vi "ensure_selection_matches_spots.vi"(4 "Selection and Groups in":T3[](array[typedef]), 6 "Select All (default: no)":bool, 7 "Spots":T1[](array[typedef]) {"Amplitude Correction" step=0.1; "Line Trapping"."Phase Gradient" step=0.05; "Line Trapping"."Vector"."x" step=1e-06 format="%#_6p"; "Line Trapping"."Vector"."y" step=1e-06 format="%#_6p"; "Line Trapping"."Vector"."z" step=1e-06 format="%#_6p"; "NA Position"."r" step=1e-06; "NA Position"."y" step=1e-06; "NA Position"."x" step=1e-06; "Position"."z" step=1e-06; "Position"."y" step=1e-06; "Position"."x" step=1e-06; "Phase" step=0.7753; "Intensity" step=0.1}) -> (0 "Selection and Groups out":T3[](array[typedef]), 3 "Spots (duplicate)":T1[](array[typedef]) {"Amplitude Correction" step=0.1; "Line Trapping"."Phase Gradient" step=0.05; "Line Trapping"."Vector"."x" step=1e-06 format="%#_6p"; "Line Trapping"."Vector"."y" step=1e-06 format="%#_6p"; "Line Trapping"."Vector"."z" step=1e-06 format="%#_6p"; "NA Position"."r" step=1e-06; "NA Position"."y" step=1e-06; "NA Position"."x" step=1e-06; "Position"."z" step=1e-06; "Position"."y" step=1e-06; "Position"."x" step=1e-06; "Phase" step=0.7753; "Intensity" step=0.1})   [LabVIEW 2015]
doc: "This VI checks that the lengths of the \"selection\" and \"spots\" arrays are the same. If not, the selection array is replaced with a new array, having all the groups set to 0 and all the selected flags set either to true (default) or false. This can be used to ensure consistency in case of dodgy code, or to make a VI behave sensibly when the selection isn't wired in."
uses:
  spot.ctl
  line_trapping.ctl
  selection_element.ctl
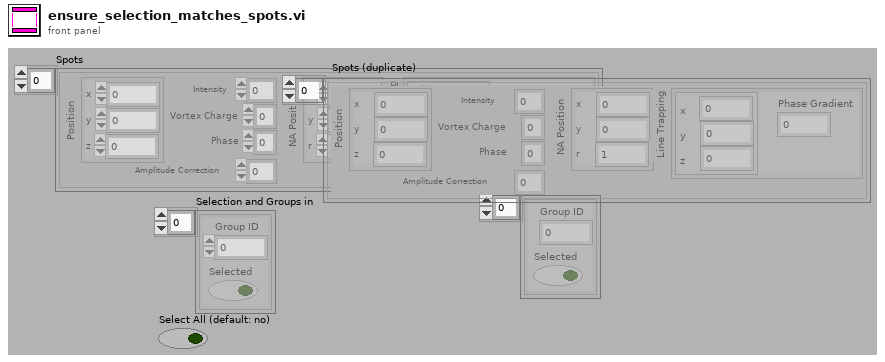
[diagram p1: front panel]
types:
  T1 = typedef "spot.ctl" = cluster{"Position":cluster{"x":dbl, "y":dbl, "z":dbl}, "Intensity":dbl, "Vortex Charge":i8, "Phase":dbl, "NA Position":cluster{"x":dbl, "y":dbl, "r":dbl}, "Line Trapping":T2, "Amplitude Correction":dbl}
  T2 = typedef "line_trapping.ctl" = cluster{"Vector":cluster{"x":dbl, "y":dbl, "z":dbl}, "Phase Gradient":dbl}
  T3 = typedef "selection_element.ctl" = cluster{"Group ID":i32, "Selected":bool}
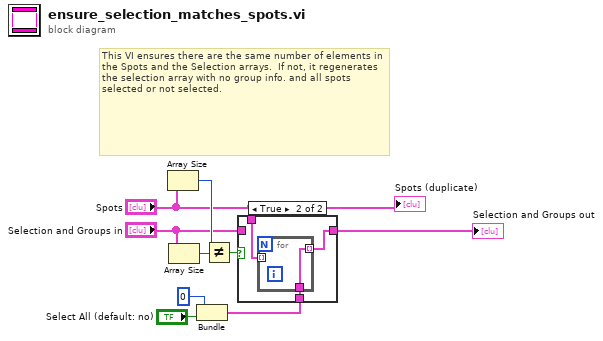
[diagram p0: block diagram]
diagram:
  # "This VI ensures there are the same number of elements in the Spots and the Selection arrays.  If not, it regenerates the selection array with no group info. and all spots selected or not selected."
  n1 = Array Size(array="Spots") -> (size(s)=w6:i32)
  n2 = Array Size(array="Selection and Groups in") -> (size(s)=w5:i32)
  n3 = Bundle(0, "Select All (default: no)"="Select All (default: no)") -> (w9:cluster{i32, "Select All (default: no)":bool})  [unwired: 1 out]
  n4 = Not Equal?(x=w6, y=w5) -> (x != y?=w1:bool)
  n5 = case shown="True" w1 {
    tunnel: "Selection and Groups in" -> [w10 _]
    tunnel: [w10 w13] -> w4
    tunnel: "Spots" -> [_ w12]
    tunnel: w9 -> [_ w11]
    frame False {
    }
    frame True {
      n6 = for {
        tunnel: [w14] -> w13 mode=indexing
        tunnel: w12 -> [_] mode=indexing
        tunnel: w11 -> [w14]
      }
    }
  }
  "Selection and Groups out" <- w4
  "Spots (duplicate)" <- "Spots"
